vi "MH_Graph_Deltas.vi"() -> ()   [LabVIEW 2019]
uses:
  <userlib>/MultiHarp150/T2Lib/MH_T2QMessage.ctl
panel:
  in  "stop":bool
  in  "WindowWidth":u32
  out "Correlations":u32[](array[numeric])
  in  "BinSize":u32
  in  "ErrorIn":errorcluster caption="entrée d'erreur (pas d'erreur)"
  out "Graph":u32[](graph)
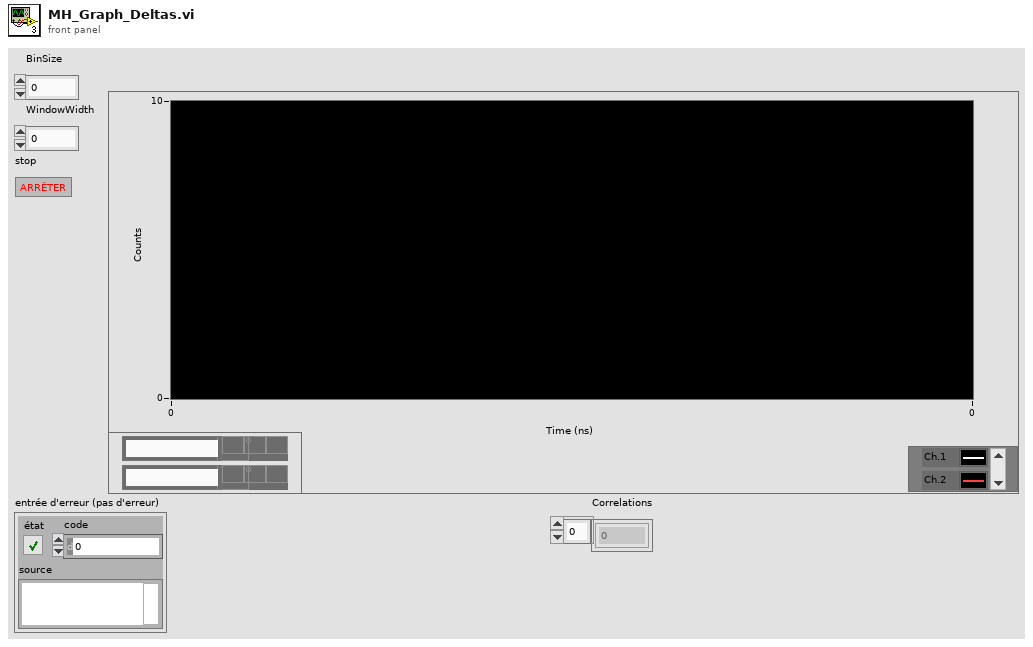
[diagram p1: front panel]
types:
  T1 = typedef "MH_T2QMessage.ctl" = cluster{"Message":string, "buffer":u32[], "Code":i32, "nactual":i32}
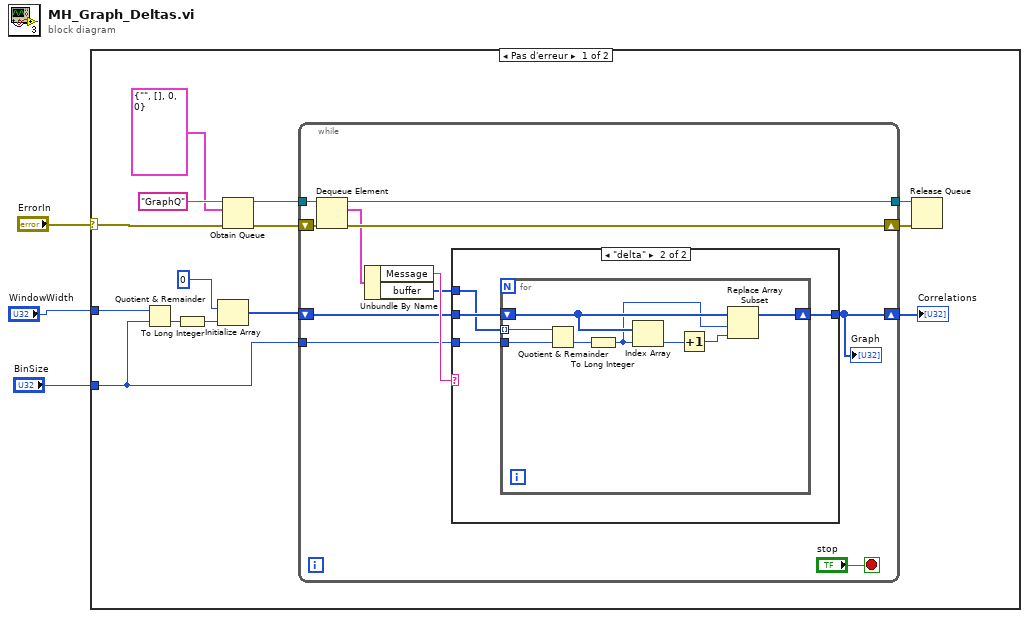
[diagram p0: block diagram]
diagram:
  n1 = case shown="Pas d'erreur" "ErrorIn" {
    selector: "ErrorIn" -> [w11 _]
    tunnel: "BinSize" -> [w8 _]
    tunnel: "WindowWidth" -> [w9 _]
    frame No Error {
      n2 = Quotient & Remainder(x=w9, y=w8) -> (floor(x/y)=w7:u32)  [unwired: 1 out]
      n3 = To Long Integer(number=w7) -> (32bit integer=w6:i32)
      n4 = Initialize Array(u32 0 ("WindowWidth"), w6) -> (w4:u32[])
      n5 = Obtain Queue(name (unnamed)="GraphQ" ("nom (aucun)"), element data type=T1 {"Message"="", "buffer"=[], "Code"=0, "nactual"=0} ("ClassQueue"), error in (no error)=w11) -> (queue out=w14:refnum<queue>, error out=w15:errorcluster)  [unwired: 2 in, 1 out]
      n6 = while {
        tunnel: w14 -> [w27]
        shift-right: [w26] -> w13
        shift-left: w15 -> [w28]
        tunnel: [w25] -> w12
        tunnel: w8 -> [w22]
        shift-right: [w19] -> w10
        shift-left: w4 -> [w21]
        stop <- "stop" stop-if-true
        n7 = Dequeue Element(queue=w27, error in (no error)=w28) -> (queue out=w25:refnum<queue>, element=w24:T1, error out=w26:errorcluster)  [unwired: 1 in, 1 out]
        n8 = Unbundle By Name(w24) -> ("Message"=w23:string, "buffer"=w20:u32[])
        n9 = case shown="\"delta\"" w23 {
          tunnel: w22 -> [_ w33]
          tunnel: w21 -> [w29 w32]
          tunnel: [w29 w31] -> w19
          tunnel: w20 -> [_ w30]
          frame "Faux", Default {
          }
          frame "delta" {
            n10 = for {
              tunnel: w30 -> [w41] mode=indexing
              tunnel: w33 -> [w40]
              shift-right: [w35] -> w31
              shift-left: w32 -> [w36]
              n11 = Quotient & Remainder(x=w41, y=w40) -> (floor(x/y)=w39:u32)  [unwired: 1 out]
              n12 = To Long Integer(number=w39) -> (32bit integer=w34:i32)
              n13 = Index Array(array=w36, index=w34) -> (element=w38:u32)
              n14 = Increment(x=w38) -> (x+1=w37:u32)
              n15 = Replace Array Subset(array=w36, new element=w37, index=w34) -> (w35:u32[])
            }
          }
        }
        "Graph" <- w19
      }
      "Correlations" <- w10
      n16 = Release Queue(queue=w12, error in (no error)=w13) -> ()  [unwired: 1 in, 3 out]
    }
    frame Error {
    }
  }
